vi "Function.vi"(8 "error in (no error)":errorcluster, 10 "Numeric":dbl, 11 "Two Terminal in":refnum<class "Not Equal 0_DBL.lvclass">) -> (0 "error out":errorcluster, 2 "Result":bool, 3 "Two Terminal out":refnum<class "Not Equal 0_DBL.lvclass">)   [LabVIEW 2021, in "Not Equal 0_DBL.lvclass"]
uses:
  Not Equal 0_DBL.lvclass
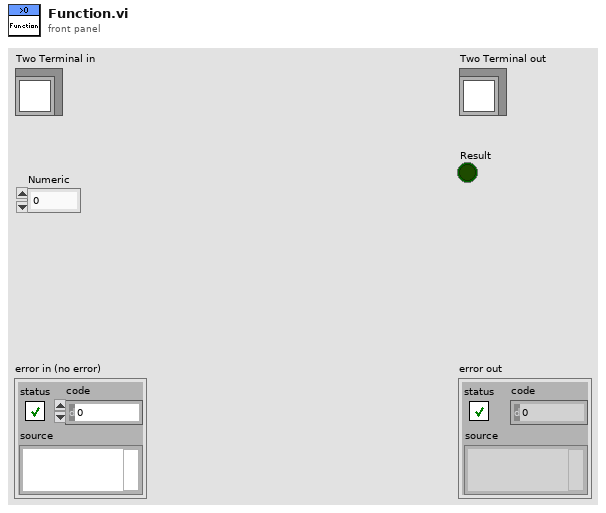
[diagram p1: front panel]
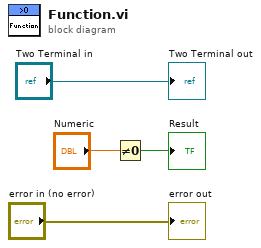
[diagram p0: block diagram]
diagram:
  n1 = Not Equal To 0?(x="Numeric") -> (x != 0?=→"Result":bool)
  "error out" <- "error in (no error)"
  "Two Terminal out" <- "Two Terminal in"
